vi "Connection Settings.vi"(8 "error in (no error)":errorcluster, 11 "Configuration in":refnum<class "Configuration.lvclass">) -> (0 "error out":errorcluster, 3 "Configuration out":refnum<class "Configuration.lvclass">)   [LabVIEW 2013, in "Client Controller.lvlib" / "Client Config.lvclass"]
uses:
  Client Config.lvclass
  <userlib>/Configuration Dialog Actor/Configuration.lvclass
  Client Config.lvclass/Client Config.ctl
panel:
  in  "Port":i32
  in  "IP Address of Server":string
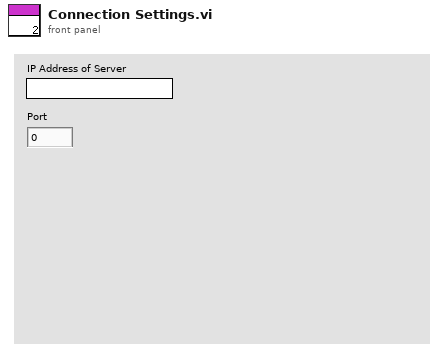
[diagram p1: front panel]
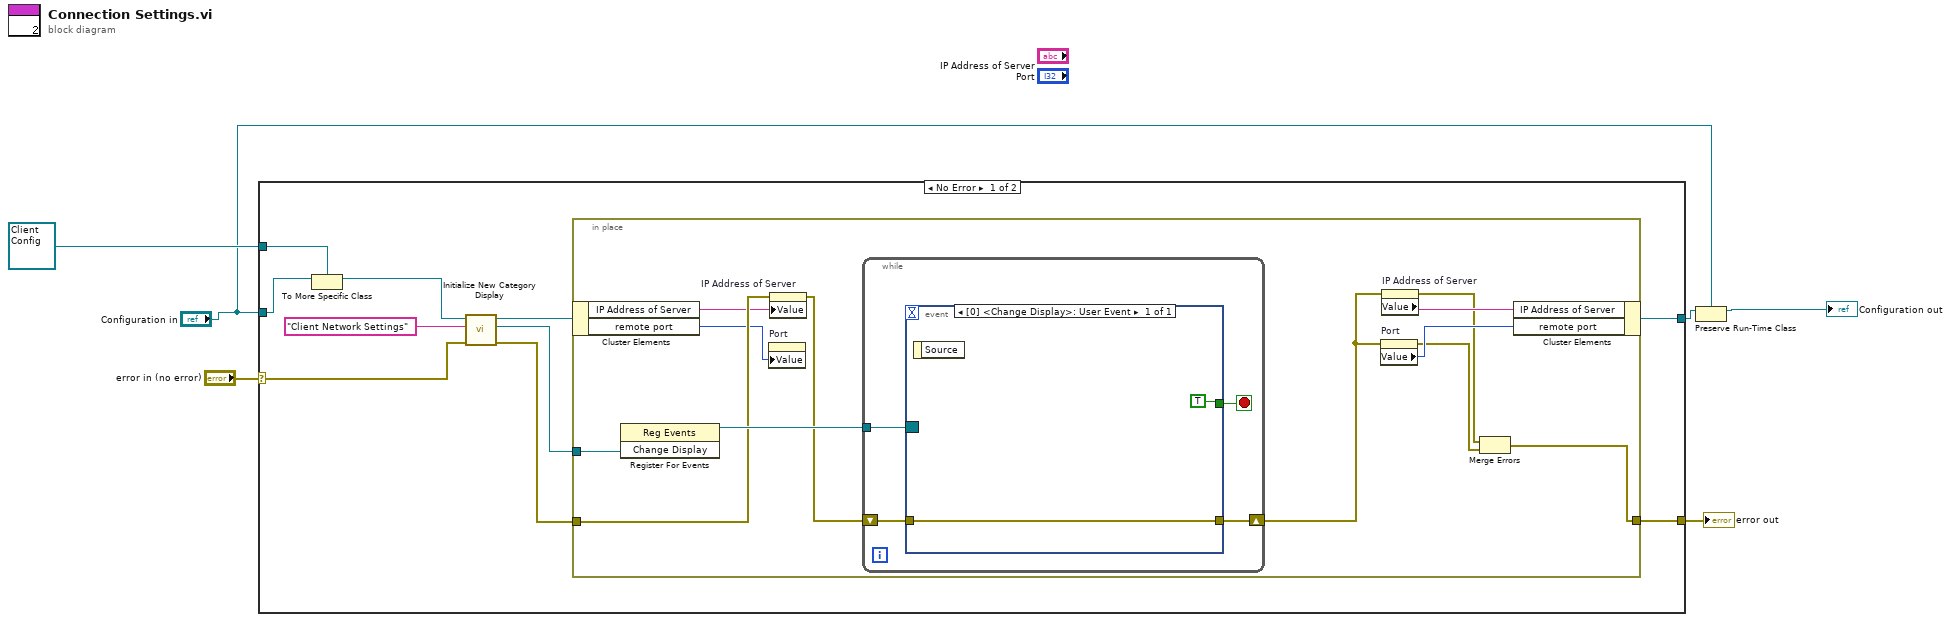
[diagram p0: block diagram]
diagram:
  n1 = case shown="No Error" "error in (no error)" {
    selector: "error in (no error)" -> [w12 w36]
    tunnel: [w11 w35] -> w2
    tunnel: [w14 w36] -> w6
    tunnel: "Configuration in" -> [w9 w35]
    tunnel: refnum<class "Client Config.lvclass"> refnum ("Client Controller.lvlib:Client Config.lvclass") -> [w7 _]
    frame No Error {
      n2 = To More Specific Class(target class=w7, reference=w9) -> (specific class reference=w8:refnum<class "Client Config.lvclass">)  [unwired: 1 in, 1 out]
      n3 = call <userlib>:"Initialize New Category Display.vi"("error in (no error)"=w12, "Name to Display"="Client Network Settings", "Configuration in"=w8) -> ("error out"=w15:errorcluster, "Change Display"=w16:refnum<user-event>, "Configuration Out"=w10:refnum<class "Client Config.lvclass">)  [unwired: 6 in]
      n4 = in-place {
        in-place-border: w16 -> [w28]
        in-place-border: w15 -> [w26]
        in-place-border: [w19] -> w14
        n5 = in-place-cluster #1(w10) -> ("IP Address of Server"=w25:string, "remote port"=w24:u16)
        n6 = register-events(w28) -> (reference out=w27:refnum<event-registration>)  [unwired: 2 in, 1 out]
        n7 = property on="Port" class="DigNum (strict)"("Value"=w24) -> ()  [unwired: 2 in, 2 out]
        n8 = property on="IP Address of Server" class="Str"(error in=w26, "Value"=w25) -> (error out=w23:errorcluster)  [unwired: 1 in, 1 out]
        n9 = while {
          tunnel: w27 -> [w31]
          shift-right: [w30] -> w22
          shift-left: w23 -> [w29]
          stop <- w32 stop-if-true
          n10 = event shown="[0] <Change Display>: User Event" {
            selector: w31 -> [_]
            dyn-events: _ -> [_]
            timeout: _ -> [_]
            tunnel: [TRUE] -> w32
            tunnel: [w33] -> w30
            tunnel: w29 -> [w33]
            event User Event {
              n11 = event-data() -> ()  [unwired: 1 in, 1 out]
            }
          }
        }
        n12 = property on="Port" class="DigNum (strict)"(error in=w22) -> (error out=w17:errorcluster, "Value"=w21:i32)  [unwired: 1 in, 1 out]
        n13 = property on="IP Address of Server" class="Str"(error in=w22) -> (error out=w18:errorcluster, "Value"=w20:string)  [unwired: 1 in, 1 out]
        n14 = Merge Errors(w18, w17) -> (w19:errorcluster)
        n15 = in-place-cluster #1("IP Address of Server"=w20, "remote port"=w21) -> (w11:refnum<class "Client Config.lvclass">)
      }
    }
    frame Error {
    }
  }
  "error out" <- w6
  n16 = Preserve Run-Time Class(object in=w2, 2:"Configuration in") -> (object out=→"Configuration out":refnum<class "Configuration.lvclass">)  [unwired: 1 in, 1 out]
